vi "Read Nb Channel.vi"(8 "error in (no error)":errorcluster, 11 "Class LED Analyser FEASA in":refnum<class "Class LED Analyser FEASA.lvclass">) -> (0 "error out":errorcluster, 2 "Nb Channel":u16, 3 "Class LED Analyser FEASA out":refnum<class "Class LED Analyser FEASA.lvclass">)   [LabVIEW 2020, in "Library Instrument & Equipement.lvlib" / "Library LED Analyser.lvlib" / "Class LED Analyser FEASA.lvclass"]
uses:
  Class LED Analyser FEASA.lvclass
  Class LED Analyser FEASA.lvclass/Class LED Analyser FEASA.ctl
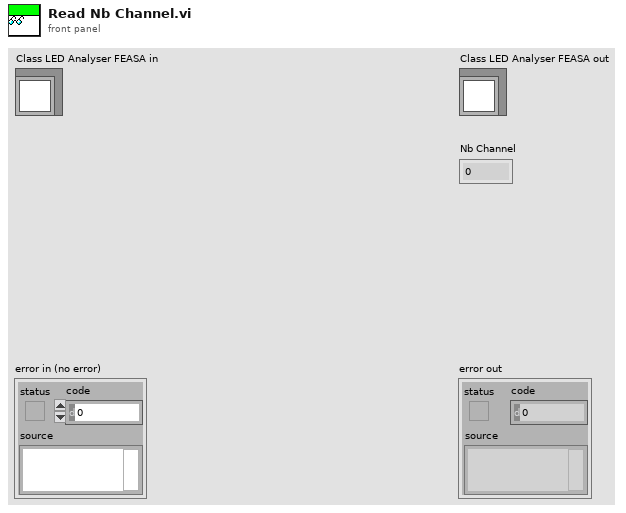
[diagram p1: front panel]
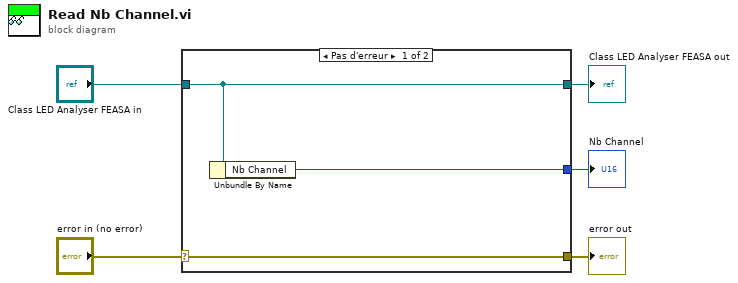
[diagram p0: block diagram]
diagram:
  n1 = case shown="Pas d'erreur" "error in (no error)" {
    selector: "error in (no error)" -> [w8 w9]
    tunnel: [w8 w9] -> w4
    tunnel: [w7 w10] -> w2
    tunnel: "Class LED Analyser FEASA in" -> [w7 w10]
    tunnel: [w6 _] -> w1
    frame No Error {
      n2 = Unbundle By Name(w7) -> ("Nb Channel"=w6:u16)
    }
    frame Error {
    }
  }
  "error out" <- w4
  "Class LED Analyser FEASA out" <- w2
  "Nb Channel" <- w1
